vi "Incar_wait.vi"() -> ()   [LabVIEW 2024]
uses:
  Incar_state.ctl
  MsgCluster.ctl
panel:
  out "Numeric":i32
  out "t0":dbl format="%_19f"
  out "now":dbl format="%_19f"
  out "Waveform Chart":dbl(graph)
  out "x-y":i32
  out "counter":bool
  out "start":i32
  out "end":i32
  out "x+y":dbl
  out "Eventループ終了":bool
  out "consumer1終了した":bool
  out "Data":dbl[](array[numeric])
  out "path 5":string
  out "MsgType 2":T1
  out "path 4":string
  out "動画終了フラグ":bool
  out "解析開始フラグ":bool
  in  "計測開始":bool
  out "element":T2
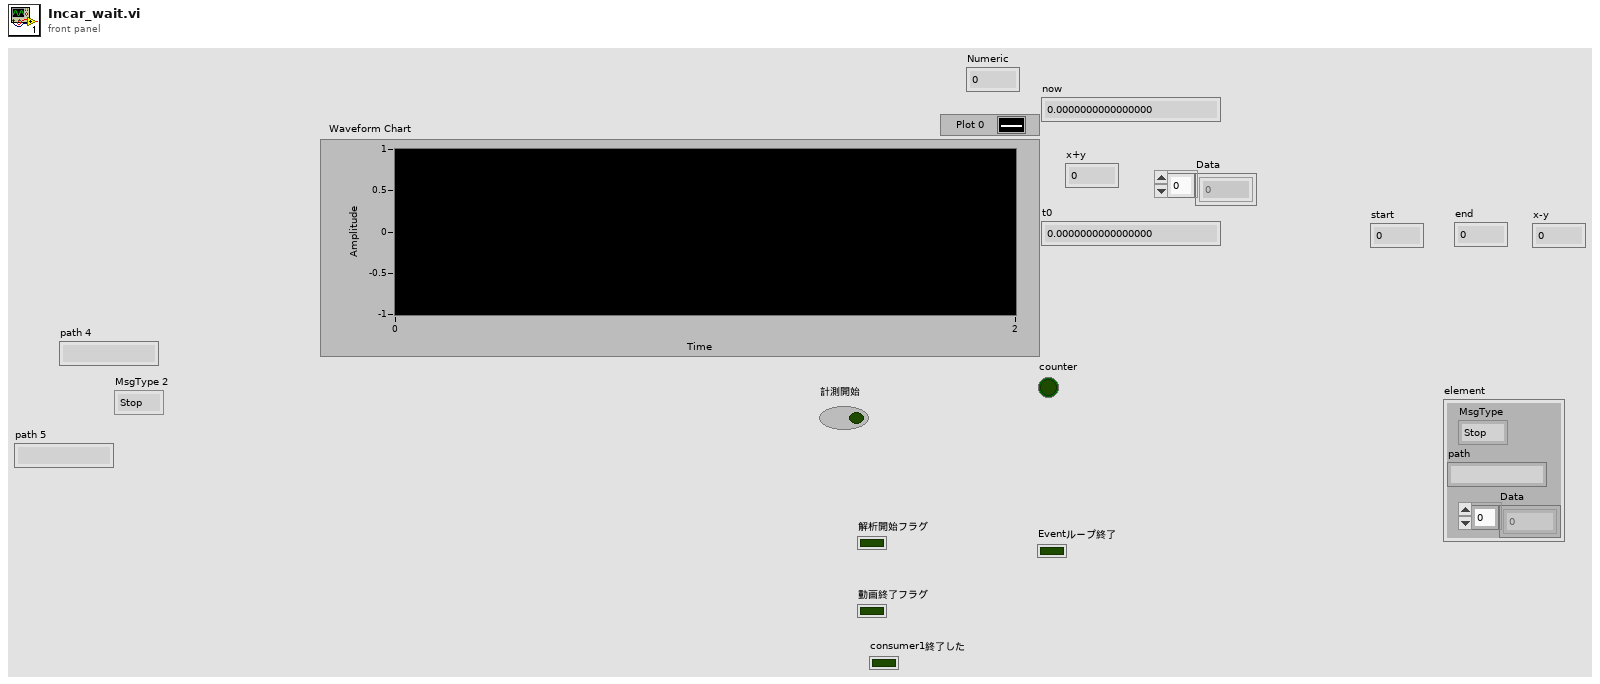
[diagram p1: front panel]
types:
  T1 = typedef "MsgCluster.ctl" = enum16{"Stop", "Start", "Data"}
  T2 = cluster{"MsgType":T1, "path":string, "Data":dbl[]}
  T3 = typedef "Incar_state.ctl" = enum16{"初期化", "待機", "練習", "計測", "解析", "全終了"}
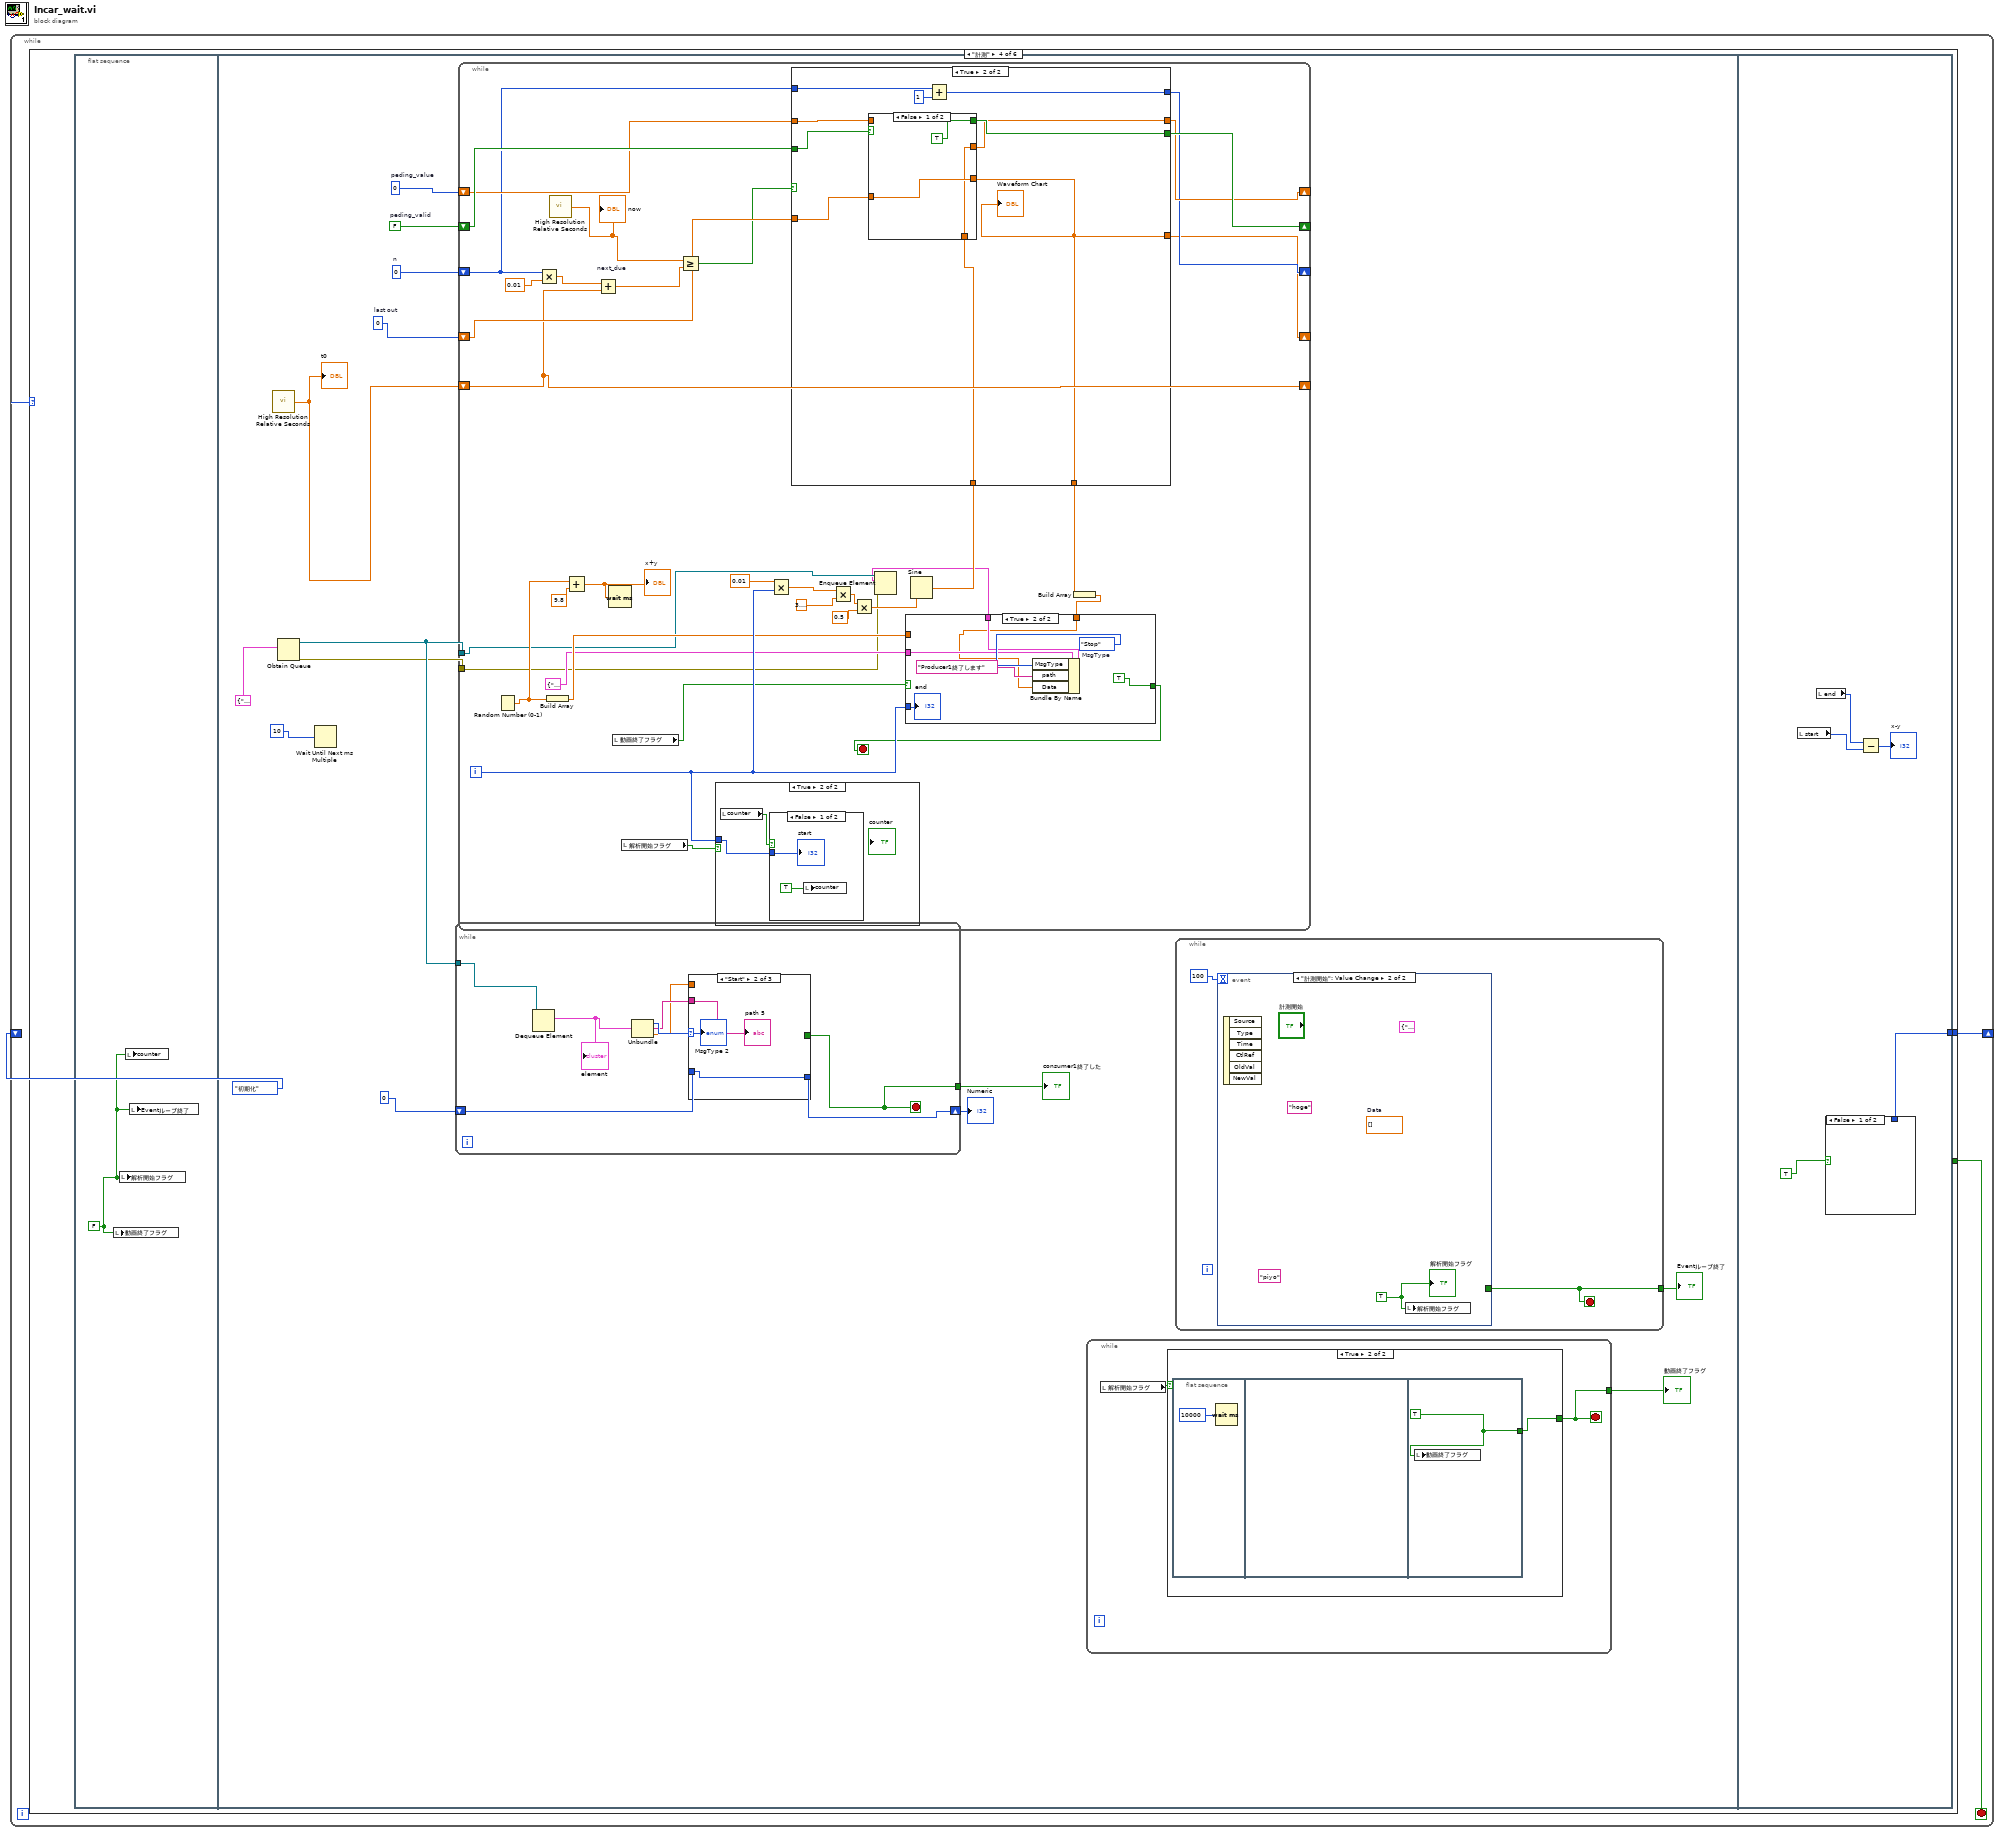
[diagram p0: block diagram]
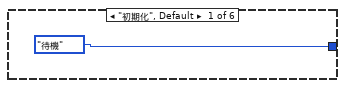
[diagram p2: hidden frame]
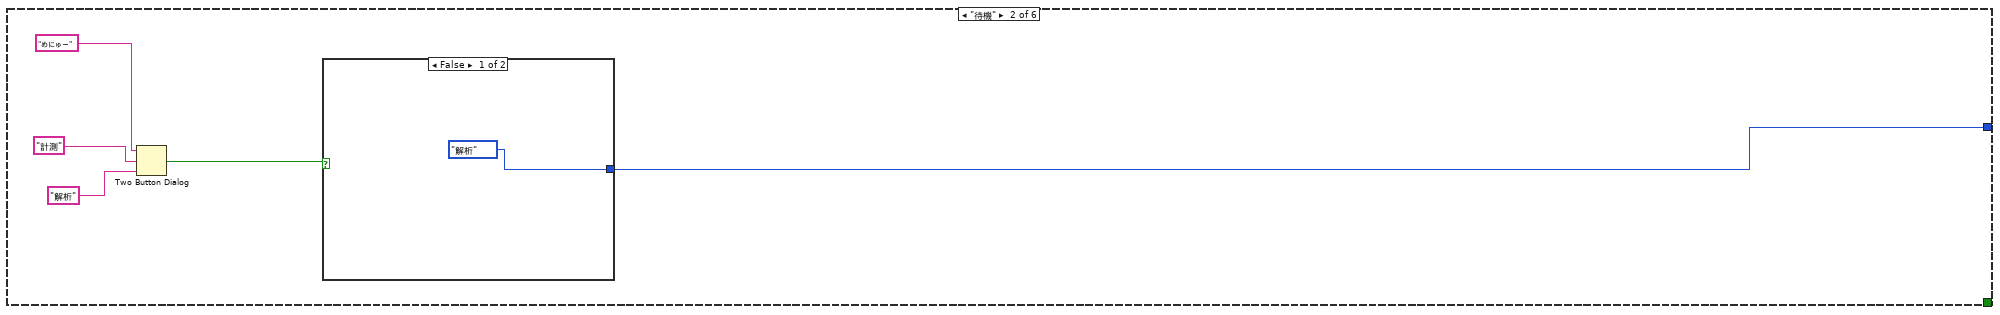
[diagram p3: hidden frame]
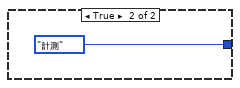
[diagram p4: hidden frame]
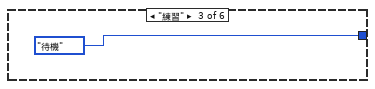
[diagram p5: hidden frame]
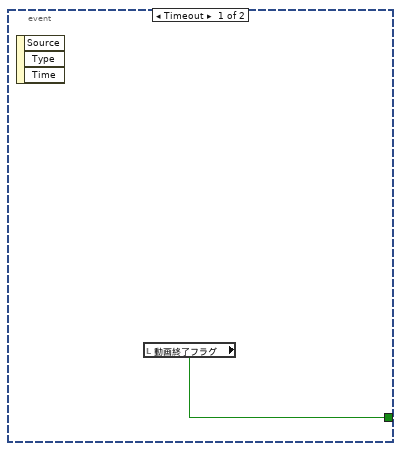
[diagram p7: hidden frame]
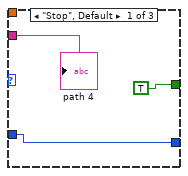
[diagram p8: hidden frame]
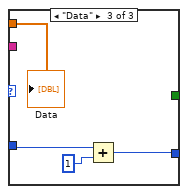
[diagram p9: hidden frame]
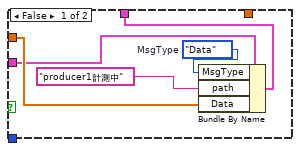
[diagram p10: hidden frame]
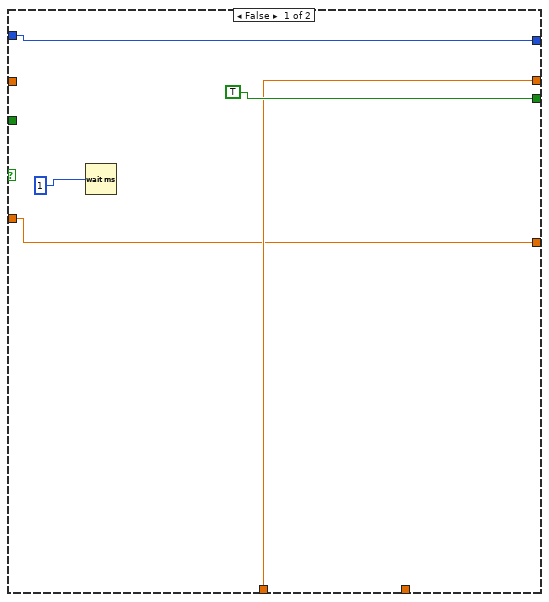
[diagram p11: hidden frame]
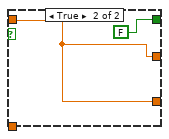
[diagram p12: hidden frame]
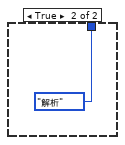
[diagram p15: hidden frame]
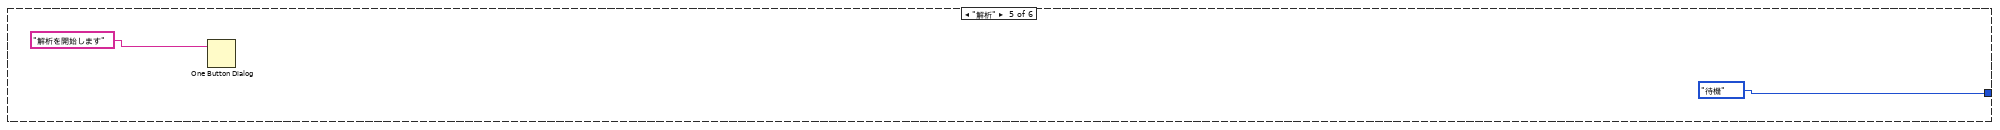
[diagram p16: hidden frame]
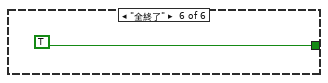
[diagram p17: hidden frame]
diagram:
  n1 = while {
    shift-right: [w3] -> _
    shift-left: Incar_state."初期化" -> [w4]
    stop <- w2 stop-if-true
    n2 = case shown="\"計測\"" w4 {
      tunnel: [Incar_state."待機" w7 Incar_state."待機" w14 Incar_state."待機" _] -> w3
      tunnel: [_ _ _ _ _ TRUE] -> w2
      frame "初期化", Default {
      }
      frame "待機" {
        n3 = Two Button Dialog(message="めにゅー", 1:"解析", 2:"計測") -> (T button?=w8:bool)
        n4 = case shown="False" w8 {
          tunnel: [Incar_state."解析" Incar_state."計測"] -> w7
          frame False {
          }
          frame True {
          }
        }
      }
      frame "練習" {
      }
      frame "計測" {
        n5 = flat-sequence {
          tunnel: [w132] -> w14
          frame #0 {
            w15 = FALSE
            n6 = local write "動画終了フラグ"(w15) -> ()
            n7 = local write "解析開始フラグ"(w15) -> ()
            n8 = local write "counter"(w15) -> ()
            n9 = local write "Eventループ終了"(w15) -> ()
          }
          frame #1 {
            w18 = 0  # peding_value
            w19 = FALSE  # peding_valid
            w20 = 0  # n
            w22 = 0  # last out
            n10 = call <vilib>:"High Resolution Relative Seconds.vi"() -> ("relative seconds"=w21:dbl)
            "t0" <- w21
            n11 = Obtain Queue(element data type=T2 {"MsgType"=enum."Stop", "path"="", "Data"=[]}) -> (queue out=w28:refnum<queue>, error out=w27:errorcluster)  [unwired: 4 in, 1 out]
            n12 = Wait Until Next ms Multiple(millisecond multiple=10) -> ()  [unwired: 1 out]
            n13 = while {
              tunnel: w28 -> [w46]
              tunnel: [w41] -> w26
              shift-right: [w39] -> w16
              shift-left: 0 -> [w40]
              stop <- w41 stop-if-true
              n14 = Dequeue Element(queue=w46) -> (element=w43:T2)  [unwired: 2 in, 3 out]
              "element" <- w43
              n15 = Unbundle(w43) -> ("MsgType"=w45:T1, "path"=w44:string, "Data"=w42:dbl[])
              n16 = case shown="\"Start\"" w45 {
                selector: w45 -> [_ w51 _]
                tunnel: w44 -> [w49 w52 _]
                tunnel: [TRUE _ _] -> w41
                tunnel: w42 -> [_ _ w56]
                tunnel: w40 -> [w47 w50 w55]
                tunnel: [w47 w50 w54] -> w39
                frame "Stop", Default {
                  "path 4" <- w49
                }
                frame "Start" {
                  "path 5" <- w52
                  "MsgType 2" <- w51
                }
                frame "Data" {
                  n17 = Add(x=w55, y=1) -> (x+y=w54:i32)
                  "Data" <- w56
                }
              }
            }
            "consumer1終了した" <- w26
            "Numeric" <- w16
            n18 = while {
              tunnel: w28 -> [w59]
              tunnel: w27 -> [w57]
              shift-right: [w73] -> _
              shift-left: w21 -> [w73]
              shift-right: [w74] -> _
              shift-left: w22 -> [w78]
              shift-right: [w75] -> _
              shift-left: w20 -> [w76]
              shift-right: [w79] -> _
              shift-left: w19 -> [w81]
              shift-right: [w77] -> _
              shift-left: w18 -> [w80]
              i -> [w66]
              stop <- w62 stop-if-true
              n19 = Random Number (0-1)() -> (number: 0 to 1=w90:dbl)
              n20 = Multiply(x=w76, y=0.01) -> (x*y=w70:dbl)
              n21 = Build Array(w90) -> (w64:dbl[])
              n22 = call <vilib>:"High Resolution Relative Seconds.vi"() -> ("relative seconds"=w68:dbl)
              "now" <- w68
              n23 = Add(x=w90, y=9.8) -> (x+y=w91:dbl)
              "x+y" <- w91
              n24 = Add "next_due"(x=w70, y=w73) -> (x+y=w67:dbl)
              n25 = Wait (ms)(milliseconds to wait=w91) -> ()  [unwired: 1 out]
              n26 = local read "動画終了フラグ"() -> (w65:bool)
              n27 = local read "解析開始フラグ"() -> (w88:bool)
              n28 = Greater Or Equal?(x=w68, y=w67) -> (x >= y?=w69:bool)
              n29 = case shown="True" w88 {
                tunnel: w66 -> [_ w124]
                frame False {
                }
                frame True {
                  n30 = local read "counter"() -> (w125:bool)
                  n31 = case shown="False" w125 {
                    tunnel: w124 -> [w127 _]
                    frame False {
                      n32 = local write "counter"(TRUE) -> ()
                      "start" <- w127
                    }
                    frame True {
                    }
                  }
                }
              }
              n33 = Multiply(x=0.01, y=w66) -> (x*y=w86:dbl)
              n34 = Multiply(x=w86, y=3.141592653589793) -> (x*y=w84:dbl)
              n35 = Multiply(x=w84, y=0.5) -> (x*y=w82:dbl)
              n36 = Sine(x=w82) -> (sin(x)=w72:dbl)
              n37 = case shown="True" w69 {
                tunnel: w81 -> [_ w118]
                tunnel: w80 -> [_ w117]
                tunnel: [TRUE w116] -> w79
                tunnel: w78 -> [w104 w115]
                tunnel: [w106 w114] -> w77
                tunnel: w72 -> [w106 w113]
                tunnel: w76 -> [w105 w112]
                tunnel: [w105 w110] -> w75
                tunnel: [w104 w109] -> w74
                tunnel: [_ w109] -> w61
                frame False {
                  n38 = Wait (ms)(milliseconds to wait=1) -> ()  [unwired: 1 out]
                }
                frame True {
                  n39 = case shown="False" w118 {
                    tunnel: w117 -> [_ w122]
                    tunnel: [TRUE FALSE] -> w116
                    tunnel: [w121 w122] -> w109
                    tunnel: w115 -> [w121 _]
                    tunnel: [w119 w122] -> w114
                    tunnel: w113 -> [w119 _]
                    frame False {
                    }
                    frame True {
                    }
                  }
                  "Waveform Chart" <- w109
                  n40 = Add(x=w112, y=1) -> (x+y=w110:i32)
                }
              }
              n41 = Build Array(w61) -> (w60:dbl[])
              n42 = case shown="True" w65 {
                tunnel: w64 -> [w94 _]
                tunnel: [w92 w101] -> w58
                tunnel: T2 {"MsgType"=enum."Stop", "path"="", "Data"=[]} -> [w93 w100]
                tunnel: [_ TRUE] -> w62
                tunnel: w66 -> [_ w98]
                tunnel: w60 -> [_ w97]
                frame False {
                  w95 = MsgCluster."Data"  # MsgType
                  n43 = Bundle By Name(cluster=w93, "MsgType"=w95, "path"="producer1計測中", "Data"=w94) -> (w92:T2)
                }
                frame True {
                  w102 = MsgCluster."Stop"  # MsgType
                  n44 = Bundle By Name(cluster=w100, "MsgType"=w102, "path"="Producer1終了します", "Data"=w97) -> (w101:T2)
                  "end" <- w98
                }
              }
              n45 = Enqueue Element(queue=w59, element=w58, error in (no error)=w57) -> ()  [unwired: 1 in, 3 out]
            }
            n46 = while {
              tunnel: [w30] -> w25
              stop <- w30 stop-if-true
              n47 = local read "解析開始フラグ"() -> (w31:bool)
              n48 = case shown="True" w31 {
                tunnel: [_ w32] -> w30
                frame False {
                }
                frame True {
                  n49 = flat-sequence {
                    tunnel: [w34] -> w32
                    frame #0 {
                      n50 = Wait (ms)(milliseconds to wait=10000) -> ()  [unwired: 1 out]
                    }
                    frame #1 {
                    }
                    frame #2 {
                      w34 = TRUE
                      n51 = local write "動画終了フラグ"(w34) -> ()
                    }
                  }
                }
              }
            }
            "動画終了フラグ" <- w25
            n52 = while {
              tunnel: [w36] -> w24
              stop <- w36 stop-if-true
              n53 = event shown="[1] \"計測開始\": Value Change" {
                selector: _ -> [_ _]
                dyn-events: _ -> [_ _]
                timeout: 100 -> [_ _]
                tunnel: [w37 _] -> w36
                event Timeout {
                  n54 = event-data() -> ()  [unwired: 1 in, 3 out]
                  n55 = local read "動画終了フラグ"() -> (w37:bool)
                }
                event "計測開始": Value Change {
                  w38 = TRUE
                  (unwired) "piyo"
                  (unwired) T2 {"MsgType"=enum."Stop", "path"="", "Data"=[]}
                  (unwired) dbl[] []  # Data
                  (unwired) "hoge"
                  n56 = event-data() -> ()  [unwired: 1 in, 6 out]
                  n57 = local write "解析開始フラグ"(w38) -> ()
                  "解析開始フラグ" <- w38
                }
              }
            }
            "Eventループ終了" <- w24
          }
          frame #2 {
            n58 = local read "start"() -> (w129:i32)
            n59 = local read "end"() -> (w130:i32)
            n60 = case shown="False" TRUE {
              tunnel: [_ Incar_state."解析"] -> w132
              frame False {
              }
              frame True {
              }
            }
            n61 = Subtract(x=w130, y=w129) -> (x-y=→"x-y":i32)
          }
        }
      }
      frame "解析" {
        n62 = One Button Dialog(message="解析を開始します") -> ()  [unwired: 1 in, 1 out]
      }
      frame "全終了" {
      }
    }
  }
